vi "Read Bytes Sync.vi"(8 "error in (no error)":errorcluster, 10 "len":i32, 11 "RTL-SDR in":refnum<class "Session.lvclass">) -> (0 "error out":errorcluster, 2 "buf":u8[](array[numeric]), 3 "RTL-SDR out":refnum<class "Session.lvclass">)   [LabVIEW 2020, in "RTL-SDR.lvlib" / "Session.lvclass"]
uses:
  Session.lvclass
  C:/dev/IlluminatedG/lv-rtl-sdr/lib/librtlsdr.dll
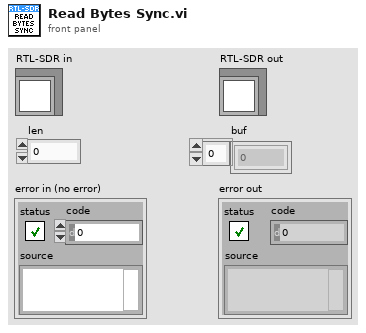
[diagram p1: front panel]
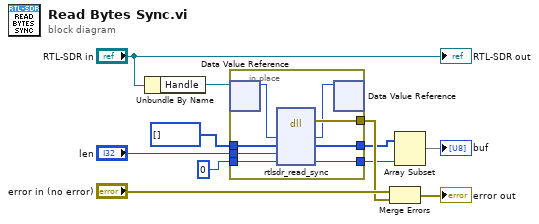
[diagram p0: block diagram]
diagram:
  n1 = Unbundle By Name("RTL-SDR in") -> ("Handle"=w1:refnum<data-value>)
  n2 = in-place {
    in-place-border: [w19] -> w7
    in-place-border: [w18] -> w6
    in-place-border: [w17] -> w5
    in-place-border: 0 ("n_read") -> [w16]
    in-place-border: "len" -> [w15]
    in-place-border: u8[] [] ("buf") -> [w14]
    n3 = in-place-dvr #1(w1) -> (w13:u64)  [unwired: 1 out]
    n4 = dll-call lib="C:/dev/IlluminatedG/lv-rtl-sdr/lib/librtlsdr.dll" fn="rtlsdr_read_sync"("dev"=w13, "buf"=w14, "len"=w15, "n_read"=w16) -> (error out=w19:errorcluster, "dev"=w12:u64, "buf"=w17:u8[], "n_read"=w18:i32)  [unwired: 5 in, 1 out]
    n5 = in-place-dvr #1(w12) -> ()  [unwired: 2 out]
  }
  n6 = Merge Errors("error in (no error)", w7) -> (→"error out":errorcluster)
  n7 = Array Subset(array=w5, length=w6) -> (→"buf":u8[])  [unwired: 1 in]
  "RTL-SDR out" <- "RTL-SDR in"
